vi "SwissSPAD Live_Is SS2 Dataset Scrambled.vi"(8 "Error In":errorcluster, 11 "Refnum in":T1) -> (0 "Error Out":errorcluster, 1 "Right band max":sgl, 2 "Left band max":sgl, 3 "SS2 image is scrambled":bool, 4 "Warning":string, 5 "Full-size image":bool)   [LabVIEW 2021, in "SwissSPAD Live.lvlib"]
uses:
  <vilib>/vision/Image Controls.llb/IMAQ Image.ctl
  SwissSPAD Live.lvlib
  <vilib>/vision/NI_Vision_Development_Module.lvlib
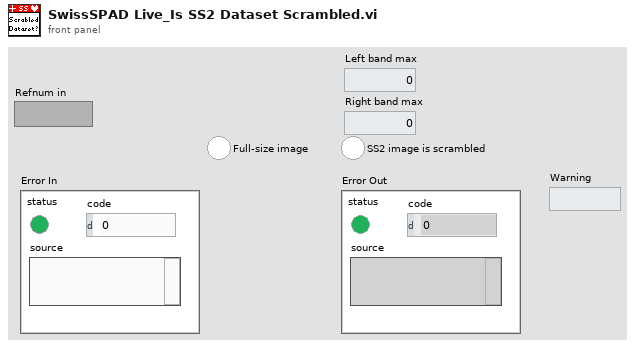
[diagram p1: front panel]
types:
  T1 = typedef "IMAQ Image.ctl" = refnum<image>
  T2 = typedef "Image Type" = u32
  T3 = cluster{"Mean Value":sgl, "Standard Variation":sgl, "Minimal Value":sgl, "Maximal Value":sgl, "Area (calibrated)":sgl, "Area (pixels)":u32, "%":sgl, "Calibration Valid":bool}[]
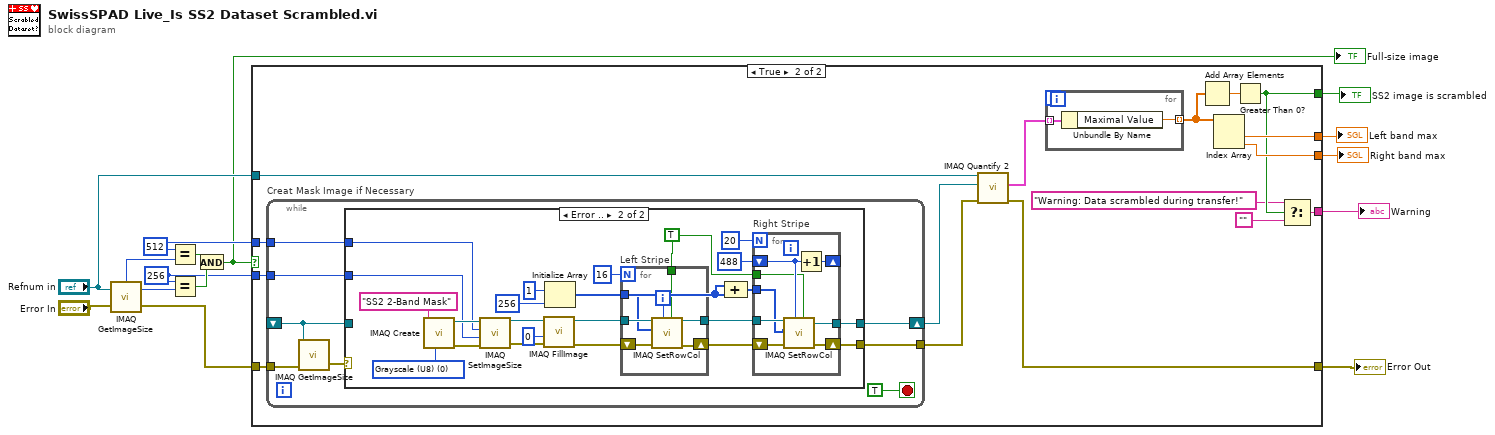
[diagram p0: block diagram]
diagram:
  w7 = 512 ("x")
  w8 = 256 ("x")
  n1 = call "IMAQ GetImageSize"("Image"="Refnum in", "error in (no error)"="Error In") -> ("Y Resolution"=w14:i32, "X Resolution"=w13:i32, "error out"=w9:errorcluster)  [unwired: 2 in]
  n2 = Equal?(x=w7, y=w13) -> (x = y?=w12:bool)
  n3 = Equal?(x=w8, y=w14) -> (x = y?=w11:bool)
  n4 = And(x=w12, y=w11) -> (x .and. y?=w3:bool)
  "Full-size image" <- w3
  n5 = case shown="True" w3 {
    tunnel: "Refnum in" -> [_ w32]
    tunnel: w9 -> [w16 w31]
    tunnel: w8 -> [_ w30]
    tunnel: w7 -> [_ w29]
    tunnel: [_ w25] -> w6
    tunnel: [_ w24] -> w5
    tunnel: [_ w21] -> w4
    tunnel: [_ w20] -> w2
    tunnel: [w16 w18] -> w1
    frame False {
    }
    frame True {
      n6 = while "Creat Mask Image if Necessary" {
        tunnel: w31 -> [w42]
        shift-right: [w39] -> w27
        shift-left: _ -> [w35]
        tunnel: w30 -> [w37]
        tunnel: w29 -> [w38]
        tunnel: [w36] -> w28
        stop <- TRUE stop-if-true
        n7 = call "IMAQ GetImageSize"("Image"=w35, "error in (no error)"=w42) -> ("error out"=w40:errorcluster)  [unwired: 2 in, 2 out]
        n8 = case shown="Error .." w40 {
          selector: w40 -> [w43 _]
          tunnel: w35 -> [w44 _]
          tunnel: [w44 w51] -> w39
          tunnel: w38 -> [_ w63]
          tunnel: w37 -> [_ w62]
          tunnel: [w43 w47] -> w36
          frame No Error {
          }
          frame Error {
            w45 = TRUE ("Row / Column (Row)")
            w67 = T2 0 items=["Grayscale (U8)", "Grayscale (I16)", "Grayscale (SGL)", "Complex (CSG)", "RGB (U32)", "HSL (U32)", "RGB (U64)", "Grayscale (U16)"] ("Image Type")
            n9 = call "IMAQ Create"("Image Name"="SS2 2-Band Mask", "Image Type"=w67) -> ("New Image"=w64:T1, "error out"=w65:errorcluster)  [unwired: 3 in]
            n10 = call "IMAQ SetImageSize"("error in (no error)"=w65, "Y Resolution"=w62, "X Resolution"=w63, "Image"=w64) -> ("error out"=w61:errorcluster, "Image Out"=w60:T1)  [unwired: 1 in]
            n11 = call "IMAQ FillImage"("error in (no error)"=w61, "Pixel Value (U8, U16, I16, Float)"=u8 0, "Image"=w60) -> ("error out"=w58:errorcluster, "Image Out"=w57:T1)  [unwired: 7 in]
            n12 = Initialize Array(u8 1 ("element"), 256 ("dimension size")) -> (w49:u8[])
            n13 = for "Left Stripe" {
              N: 16 -> [_]
              shift-right: [w77] -> w53
              shift-left: w58 -> [w82]
              tunnel: w57 -> [w81]
              tunnel: [w80] -> w52
              tunnel: w49 -> [w78]
              tunnel: w45 -> [w76]
              i -> [w79]
              n14 = call "IMAQ SetRowCol"("Row / Column (Row)"=w76, "Number"=w79, "error in (no error)"=w82, "Pixels (U8)"=w78, "Image"=w81) -> ("error out"=w77:errorcluster, "Image Out"=w80:T1)  [unwired: 5 in]
            }
            n15 = Compound Arithmetic op=unknown(w49, w49) -> (w48:u8[])
            n16 = for "Right Stripe" {
              N: 20 -> [_]
              shift-right: [w71] -> w47
              shift-left: w53 -> [w75]
              tunnel: w52 -> [w74]
              tunnel: [w73] -> w51
              tunnel: w48 -> [w72]
              shift-right: [w69] -> _
              shift-left: 488 -> [w70]
              tunnel: w45 -> [w68]
              n17 = call "IMAQ SetRowCol"("Row / Column (Row)"=w68, "Number"=w70, "error in (no error)"=w75, "Pixels (U8)"=w72, "Image"=w74) -> ("error out"=w71:errorcluster, "Image Out"=w73:T1)  [unwired: 5 in]
              n18 = Increment(x=w70) -> (x+1=w69:i32)
            }
          }
        }
      }
      n19 = call "IMAQ Quantify 2"("error in (no error)"=w28, "Image Mask"=w27, "Image"=w32) -> ("error out"=w18:errorcluster, "Region Reports"=w26:T3)  [unwired: 6 in, 1 out]
      n20 = for {
        tunnel: w26 -> [w34] mode=indexing
        tunnel: [w33] -> w23 mode=indexing
        n21 = Unbundle By Name(w34) -> ("Maximal Value"=w33:sgl)
      }
      n22 = Add Array Elements(numeric array=w23) -> (sum=w22:sgl)
      n23 = Index Array(array=w23) -> (element #1=w25:sgl, element #2=w24:sgl)  [unwired: 2 in]
      n24 = Greater Than 0?(x=w22) -> (x > 0?=w21:bool)
      n25 = Select(t="Warning: Data scrambled during transfer!" ("format string"), s=w21, f="") -> (s? t:f=w20:string)
    }
  }
  "SS2 image is scrambled" <- w4
  "Left band max" <- w6
  "Right band max" <- w5
  "Warning" <- w2
  "Error Out" <- w1
